vi "Queue.vi"(8 "error in":errorcluster, 10 "State(Get)":T1=enum."Get", 11 "VI Ref":refnum<vi>) -> (0 "error out":errorcluster, 3 "queue out":refnum<queue>)   [LabVIEW 2018, in "S2.lvclass"]
uses:
  S2.lvclass
  Queue Data.ctl
  State.ctl
  Queue.ctl
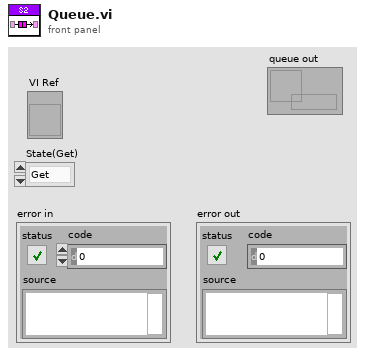
[diagram p1: front panel]
types:
  T1 = typedef "S2.lvclass/Queue.ctl" = enum16{"Create", "Get", "Destroy"}
  T2 = typedef "S2.lvclass/Queue Data.ctl" = cluster{"State":T3, "Data":variant}
  T3 = typedef "S2.lvclass/State.ctl" = enum16{"Initialize", "SetConfig", "AckAlarm", "Alarm", "Idle", "LockLid", "LowPressure", "Pressurize", "DecayTest", "Vent", "Abort", "Start", "CreateReports", "WriteToReport", "WritePressure", "Error", "Exit"}
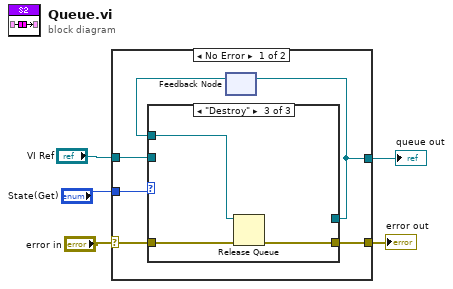
[diagram p0: block diagram]
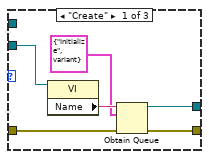
[diagram p2: hidden frame]
diagram:
  n1 = case shown="No Error" "error in" {
    selector: "error in" -> [w11 w23]
    tunnel: [w10 w23] -> w5
    tunnel: "VI Ref" -> [w9 _]
    tunnel: [w7 _] -> w2
    tunnel: "State(Get)" -> [w6 _]
    frame No Error {
      n2 = feedback #1() -> (w8:refnum<queue>)  [unwired: 1 in]
      n3 = case shown="\"Destroy\"" w6 {
        tunnel: w11 -> [w17 w19 w22]
        tunnel: [w16 w19 w20] -> w10
        tunnel: w9 -> [w15 _ _]
        tunnel: [w12 w18 _] -> w7
        tunnel: w8 -> [_ w18 w21]
        frame "Create" {
          n4 = property class="VI"(reference=w15) -> ("Name"=w14:string)  [unwired: 1 in, 2 out]
          n5 = Obtain Queue(name (unnamed)=w14, element data type=T2 {"State"=enum."Initialize", "Data"=variant}, error in (no error)=w17) -> (queue out=w12:refnum<queue>, error out=w16:errorcluster)  [unwired: 2 in, 1 out]
        }
        frame "Get", Default {
        }
        frame "Destroy" {
          n6 = Release Queue(queue=w21, error in (no error)=w22) -> (error out=w20:errorcluster)  [unwired: 1 in, 2 out]
        }
      }
      n7 = feedback-in #1(w7) -> ()
    }
    frame Error {
    }
  }
  "error out" <- w5
  "queue out" <- w2
